vi "old APU.vi"() -> ()   [LabVIEW 2015]
uses:
  <vilib>/Platform/TimedLoop/XDataNode/wakeup.ctl
  <vilib>/Platform/TimedLoop/XDataNode/XDNodeRunTimeDep.lvlib
  <vilib>/Platform/TimedLoop/XDataNode/nitl_modes.ctl
  <vilib>/Platform/TimedLoop/XDataNode/timing_clust.ctl
  <vilib>/Platform/TimedLoop/XDataNode/XDataNode.xnode
  <userlib>/_NI VeriStand FPGA Support/NI VeriStand RIO Library/Custom Device Components/Engine Simulation/Engine Simulation Globals.vi
panel:
  in  "APU.Degrees per Tick":u64
  out "APU.Crank Angle":u64
  out "APU.Cycle Angle":u64
  in  "APU.Reset":bool
  in  "APU.Increment Rate":u64
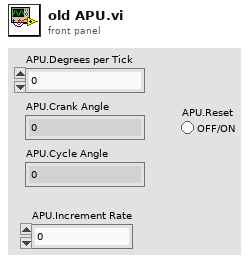
[diagram p1: front panel]
types:
  T1 = typedef "XDNodeRunTimeDep.lvlib/timing_clust.ctl" = cluster{"Expected End [f-1]":u64, "Actual End [f-1]":u64, "Finished Late? [f-1]":bool, "Expected End [i-1]":u64, "Actual End [i-1]":u64, "Finished Late? [i-1]":bool, "Expected Start [i]":u64, "Actual Start [i]":u64, "Expected Start [f]":u64, "Actual Start [f]":u64, "Source Name":string, "Structure Name":string, "Period":i64, "Deadline":i64, "Offset":i64, "Start":i64, "Priority":i32, "Timeout":i32, "Mode":T2, "Wakeup Reason":T3, "Error":errorcluster, "Source Type":string, "Secondary Source Type":string, "Global End Time":u64, "Global Start Time":u64, "Frame Duration":u64, "Iteration Duration":u64, "Assigned CPU":i32, "I/O Scan Engine Mode":u32}
  T2 = typedef "XDNodeRunTimeDep.lvlib/nitl_modes.ctl" = enum32{"No Change", "Process missed periods, maintain original phase", "Discard missed periods, maintain original phase", "Process missed periods, ignore original phase", "Discard missed periods, ignore original phase"}
  T3 = typedef "XDNodeRunTimeDep.lvlib/wakeup.ctl" = enum32{"Normal", "Aborted", "Asynchronous wakeup", "Timing source error", "Timed loop error", "Timeout"}
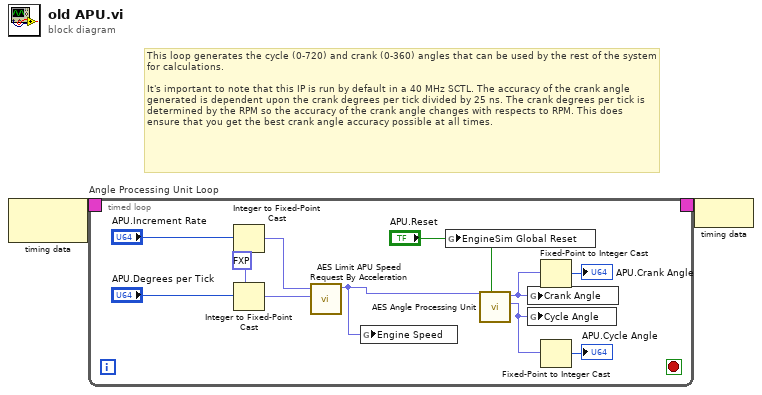
[diagram p0: block diagram]
diagram:
  # "This loop generates the cycle (0-720) and crank (0-360) angles that can be used by the rest of the system for calculations. \n\nIt's important to note that this IP is run by default in a 40 MHz SCTL. The accuracy of the crank angle generated is dependent upon the crank degrees per tick divided by 25 ns. The crank degrees per tick is determined by the RPM so the accuracy of the crank angle changes with respects to RPM. This does ensure that you get the best crank angle accuracy possible at all times."
  n1 = node-c288() -> (w2:T1)  [unwired: 1 in]
  n2 = timed-loop "Angle Processing Unit Loop" {
    timing: w2 -> [_]
    timing-out: [_] -> w1
    stop <- _ stop-if-true
    w5 = fxp<+/-,47,-4> 0.0 ("Crank.Degrees per Tick")
    n3 = Integer to Fixed-Point Cast(fixed-point type=w5, integer="APU.Increment Rate") -> (fixed-point=w4:fxp<+/-,47,-4>)
    n4 = Integer to Fixed-Point Cast(fixed-point type=w5, integer="APU.Degrees per Tick") -> (fixed-point=w7:fxp<+/-,47,-4>)
    n5 = call <userlib>:"AES Limit APU Speed Request By Acceleration.vi"("APU.Degrees per Tick in"=w7, "APU.Increment Rate"=w4) -> ("APU.Degrees per Tick out"=w3:fxp<+/-,47,-4>)  [unwired: 9 in]
    n6 = global write "Engine Simulation Globals.vi" "Engine Speed"(w3) -> ()
    n7 = global write "Engine Simulation Globals.vi" "EngineSim Global Reset"("APU.Reset") -> ()
    n8 = call <userlib>:"AES Angle Processing Unit.vi"("APU.Reset"="APU.Reset", "APU.Degrees per Tick"=w3) -> ("APU.Cycle Angle"=w9:fxp<+,61,10>, "APU.Crank Angle"=w13:fxp<+,60,9>)  [unwired: 8 in]
    n9 = global write "Engine Simulation Globals.vi" "Crank Angle"(w13) -> ()
    n10 = global write "Engine Simulation Globals.vi" "Cycle Angle"(w9) -> ()
    n11 = Fixed-Point to Integer Cast(1:w13) -> (0:→"APU.Crank Angle":u64)
    n12 = Fixed-Point to Integer Cast(1:w9) -> (0:→"APU.Cycle Angle":u64)
  }
  n13 = node-c288(w1) -> ()
